vi "Run State.vi"(8 "error in (no error)":errorcluster, 10 "Reset":bool, 11 "Stepper in":refnum<class "Stepper.lvclass">) -> (0 "error out":errorcluster, 3 "Stepper out":refnum<class "Stepper.lvclass">)   [LabVIEW 2015, in "Stepper.lvclass"]
uses:
  Stepper.lvclass
  Stepper.lvclass/Stepper.ctl
  <vilib>/ptbypt/NI_PtbyPt.lvlib
panel:
  in  "y":dbl=80000.0
  in  "sample length":i32=1
  in  "PID":cluster{"P":dbl, "I":dbl, "D":dbl}={"P"=200.0, "I"=10.0, "D"=100.0}
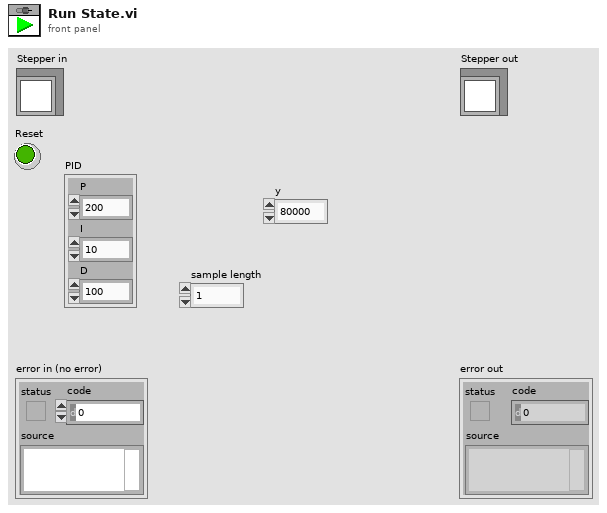
[diagram p1: front panel]
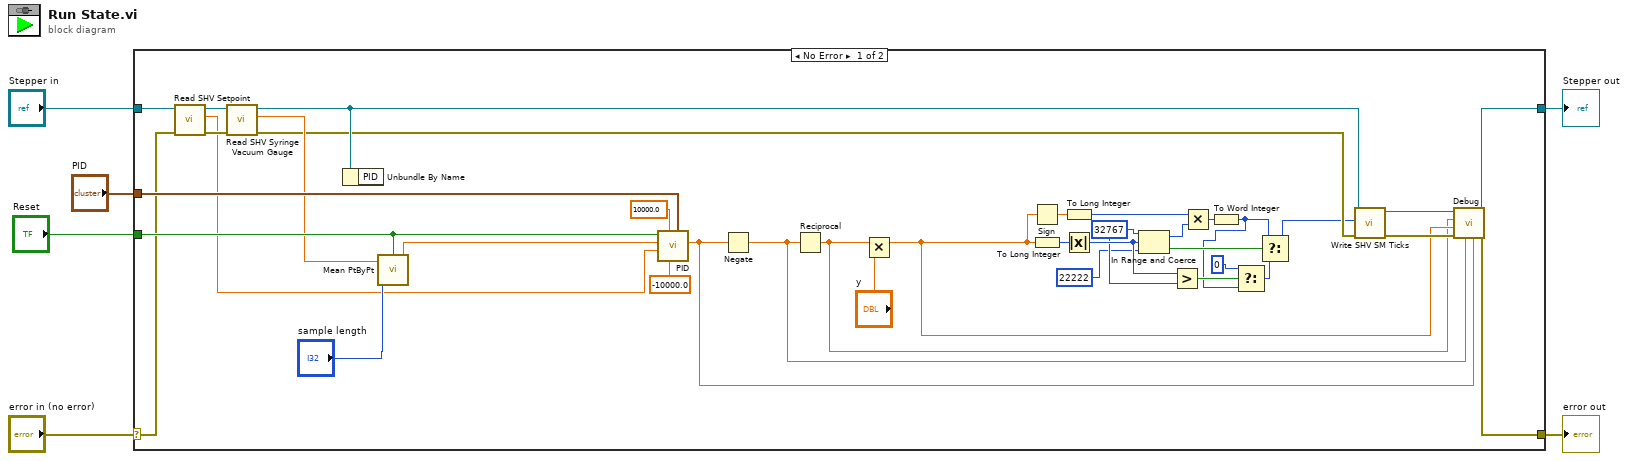
[diagram p0: block diagram]
diagram:
  n1 = case shown="No Error" "error in (no error)" {
    selector: "error in (no error)" -> [w36 w45]
    tunnel: [w30 w45] -> w5
    tunnel: [w28 w44] -> w3
    tunnel: "Stepper in" -> [w38 w44]
    tunnel: "Reset" -> [w41 _]
    tunnel: "PID" -> [w43 _]
    frame No Error {
      w13 = 32767 ("upper limit")
      n2 = call "Read SHV Setpoint.vi"("error in (no error)"=w36, "Stepper in"=w38) -> ("error out"=w35:errorcluster, "data out"=w34:dbl, "Stepper out"=w37:refnum<class "Stepper.lvclass">)  [unwired: 7 in]
      n3 = call "Read SHV Syringe Vacuum Gauge.vi"("error in (no error)"=w35, "Stepper in"=w37) -> ("error out"=w32:errorcluster, "Data"=w39:dbl, "Stepper out"=w33:refnum<class "Stepper.lvclass">)  [unwired: 7 in]
      n4 = Unbundle By Name(w33) -> ()  [unwired: 1 out]
      n5 = call <vilib>:"Mean PtByPt.vi"("x"=w39, "sample length"="sample length", "initialize"=w41) -> ("mean"=w42:dbl)  [unwired: 1 in, 1 out]
      n6 = call "PID.vi"("PID"=w43, "Lower Limit"=-10000.0, "Upper Limit (0,01)"=10000.0, "Setpoint (0,002)"=w34, "Process"=w42, "Reset"=w41) -> ("Output"=w11:dbl)  [unwired: 4 in, 1 out]
      n7 = Negate(x=w11) -> (-x=w10:dbl)
      n8 = Reciprocal(x=w10) -> (1/x=w7:dbl)
      n9 = Multiply(x=w7, y="y") -> (x*y=w8:dbl)
      n10 = Sign(1:w8) -> (0:w23:dbl)
      n11 = To Long Integer(number=w8) -> (32bit integer=w24:i32)
      n12 = To Long Integer(number=w23) -> (32bit integer=w22:i32)
      n13 = Absolute Value(x=w24) -> (abs(x)=w14:i32)
      n14 = In Range and Coerce(upper limit=w13, x=w14, lower limit=22222) -> (coerced(x)=w18:i32, In Range?=w20:bool)
      n15 = Greater?(x=w14, y=w13) -> (0:w19:bool)
      n16 = Multiply(x=w22, y=w18) -> (x*y=w21:i32)
      n17 = To Word Integer(number=w21) -> (16bit integer=w15:i16)
      n18 = Select(t=i16 0, s=w19, f=w15) -> (s? t:f=w16:i16)
      n19 = Select(t=w15, s=w20, f=w16) -> (s? t:f=w25:i16)
      n20 = call "Write SHV SM Ticks.vi"("error in (no error)"=w32, "Ticks (0)"=w25, "Stepper in"=w33) -> ("error out"=w31:errorcluster, "Stepper out"=w29:refnum<class "Stepper.lvclass">)  [unwired: 7 in]
      n21 = call "Debug.vi"("Numeric 1"=w11, "Numeric 0"=w10, "error in (no error)"=w31, "Numeric 3"=w8, "Numeric 2"=w7, "Stepper in"=w29) -> ("error out"=w30:errorcluster, "Stepper out"=w28:refnum<class "Stepper.lvclass">)  [unwired: 4 in]
    }
    frame Error {
    }
  }
  "error out" <- w5
  "Stepper out" <- w3
